vi "2019 deep space game quality.vi"() -> (0 "Quality":enum16{"Poor", "Good", "Excellent"}(ring), 1 "Level":enum16{"Level 1", "Level 2", "Level 3"}(ring))   [LabVIEW 2018]
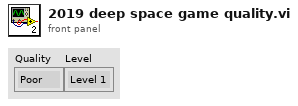
[diagram p1: front panel]
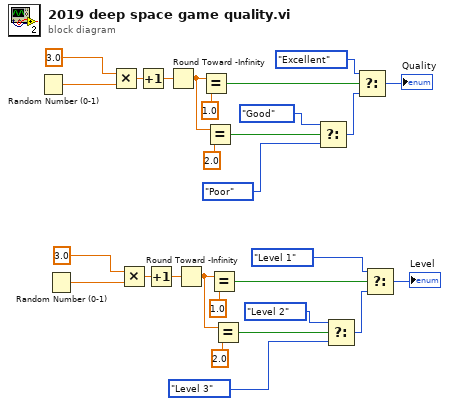
[diagram p0: block diagram]
diagram:
  n1 = Random Number (0-1)() -> (number: 0 to 1=w16:dbl)
  n2 = Random Number (0-1)() -> (number: 0 to 1=w14:dbl)
  n3 = Multiply(x=3.0, y=w16) -> (x*y=w18:dbl)
  n4 = Multiply(x=3.0, y=w14) -> (x*y=w12:dbl)
  n5 = Increment(x=w18) -> (x+1=w19:dbl)
  n6 = Increment(x=w12) -> (x+1=w11:dbl)
  n7 = Round Toward -Infinity(1:w19) -> (0:w23:dbl)
  n8 = Round Toward -Infinity(1:w11) -> (0:w7:dbl)
  n9 = Equal?(x=w23, y=1.0) -> (x = y?=w21:bool)
  n10 = Equal?(x=w23, y=2.0) -> (x = y?=w25:bool)
  n11 = Equal?(x=w7, y=1.0) -> (x = y?=w9:bool)
  n12 = Equal?(x=w7, y=2.0) -> (x = y?=w5:bool)
  n13 = Select(t=enum16{"Poor", "Good", "Excellent"}."Good", s=w25, f=enum16{"Poor", "Good", "Excellent"}."Poor") -> (s? t:f=w24:enum16{"Poor", "Good", "Excellent"})
  n14 = Select(t=enum16{"Level 1", "Level 2", "Level 3"}."Level 2", s=w5, f=enum16{"Level 1", "Level 2", "Level 3"}."Level 3") -> (s? t:f=w6:enum16{"Level 1", "Level 2", "Level 3"})
  n15 = Select(t=enum16{"Poor", "Good", "Excellent"}."Excellent", s=w21, f=w24) -> (s? t:f=→"Quality":enum16{"Poor", "Good", "Excellent"})
  n16 = Select(t=enum16{"Level 1", "Level 2", "Level 3"}."Level 1", s=w9, f=w6) -> (s? t:f=→"Level":enum16{"Level 1", "Level 2", "Level 3"})
